vi "Initiate multi-module assembly.vi"(0 "Database Entry in":refnum<class "Database Entry.lvclass">, 11 "error in (no error)":errorcluster) -> (2 "Feet check":bool, 4 "Database Entry out":refnum<class "Database Entry.lvclass">, 6 "Module?":bool, 8 "Abort out":bool, 14 "Module type out":string, 15 "error out":errorcluster)   [LabVIEW 2021, in "Database Entry.lvclass"]
uses:
  Database Entry.lvclass
  Database Entry.lvclass/Database Entry.ctl
  Components/Stack/Stack.lvclass
  <vilib>/Utility/file.llb/Read Delimited Spreadsheet (string).vi
  SubVIs/assembly_tray_region.vi
panel:
  in  "De/Select All":bool
  in  "Set default module type":bool
  out "Now assembling...":string
  in  "Abort":bool
  in  "Relative humidity":dbl
  in  "Temperature (C)":dbl
  in  "Adhesive":u16(ring) items=["Hybrid", "Transfer tape only", "Epoxy only"]
  in  "Module Type":u16(ring) items=["CMU,LD,Full,200,CuW", "CMU,LD,Full,300,CuW", "CMU,LD,Full,300,Ti", "CMU,LD,Full,200,CF", "CMU,LD,Full,300,CF"]
  in  "Operator":u16(ring) items=["jestein", "japicard", "simurthy", "shapoval", "novak", "cmumac"]
  in  "Select positions for assembly":cluster{"1":bool, "2":bool, "3":bool, "4":bool}
  in  "Submit":bool
  # "Tray Slot 1"
  # "Tray Slot 2"
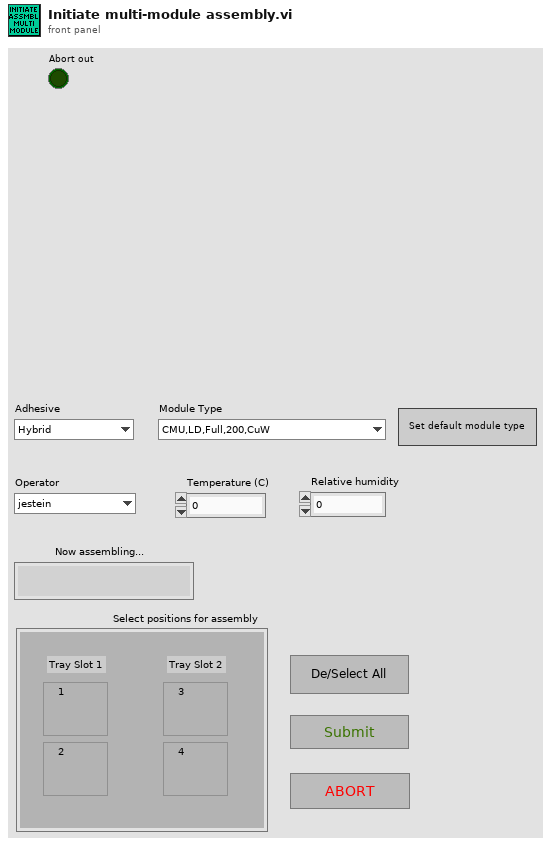
[diagram p1: front panel]
types:
  T1 = typedef "File Paths.ctl" = cluster{"Glue Pattern Folder":path, "Carrier Tray Folder":path, "Pick Up Tool Fixture Folder":path, "Components Folder":path, "Bellows Tool Offset.txt":path, "Pick Up Tool Offset.txt":path, "Dispense Tip Offset.txt":path, "Log Files":path, "Gantry Assembly Map.txt":path, "Syringe and offset map.txt":path, "Controllers Folder":path, "Local dbase config":path}
  T2 = cluster{"[0]":bool, "[1]":bool, "[2]":bool, "[3]":bool}
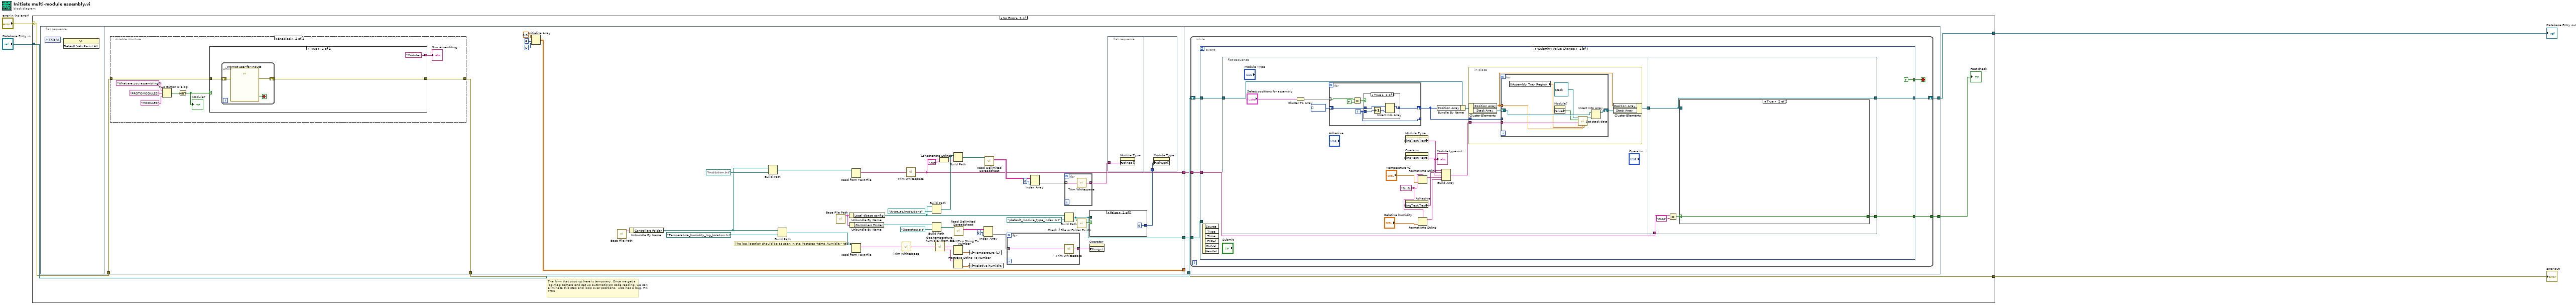
[diagram p0: block diagram]
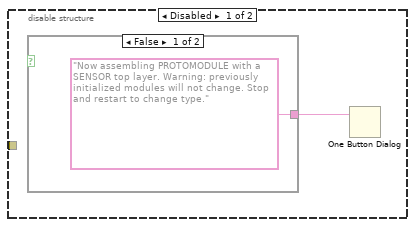
[diagram p2: hidden frame]
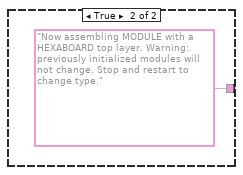
[diagram p3: hidden frame]
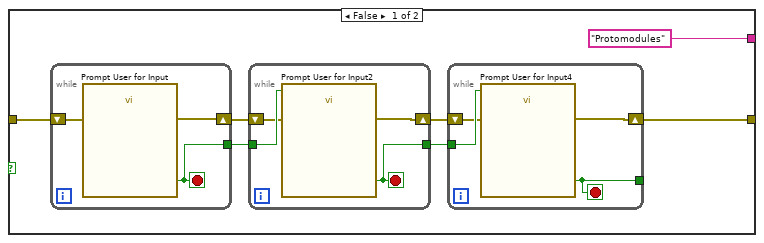
[diagram p4: hidden frame]
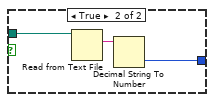
[diagram p5: hidden frame]
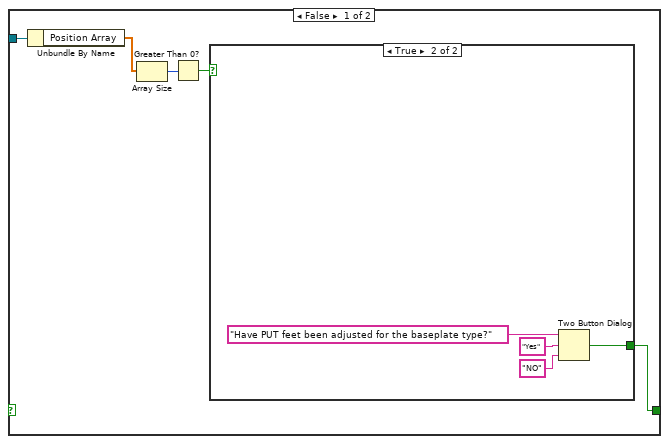
[diagram p7: hidden frame]
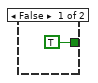
[diagram p8: hidden frame]
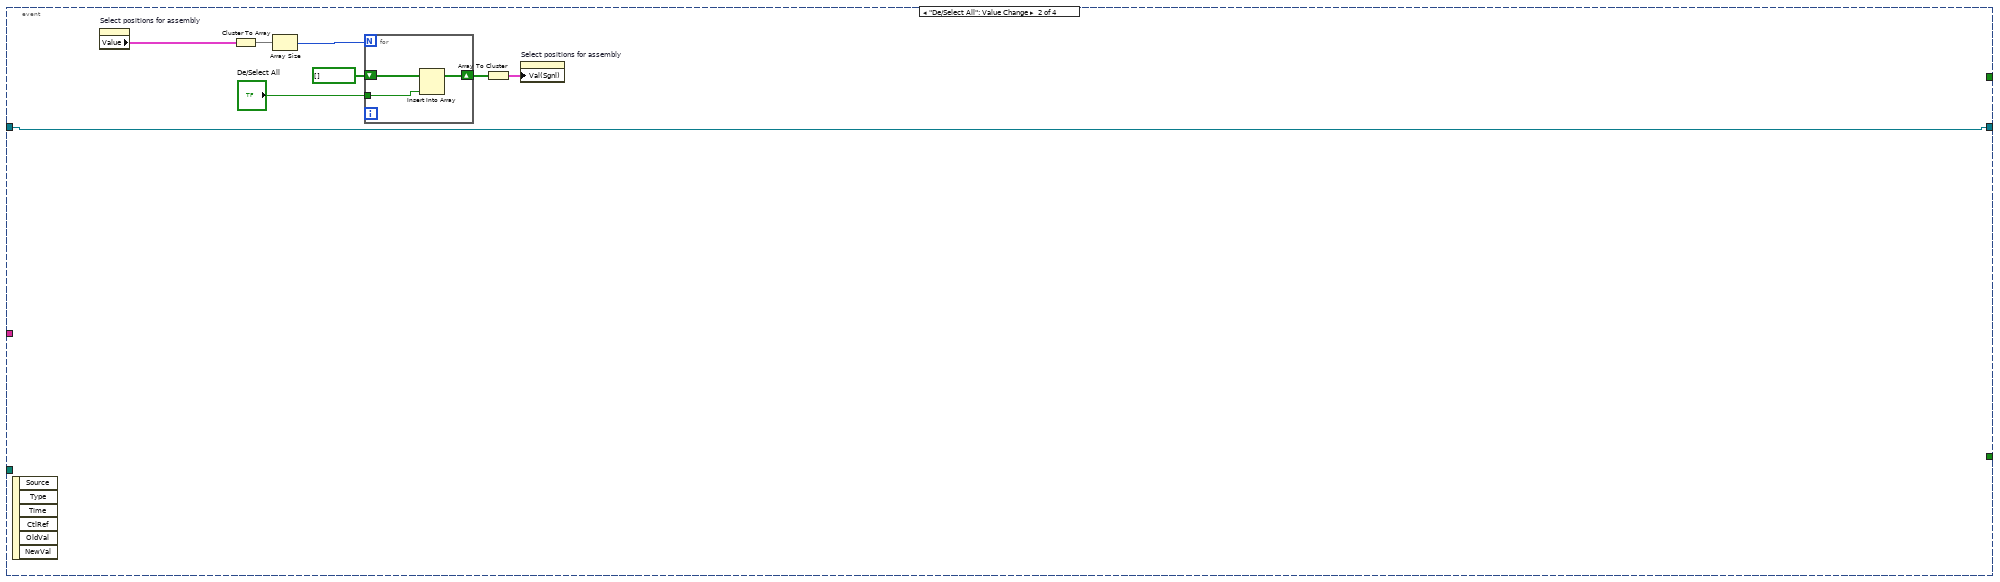
[diagram p9: hidden frame]
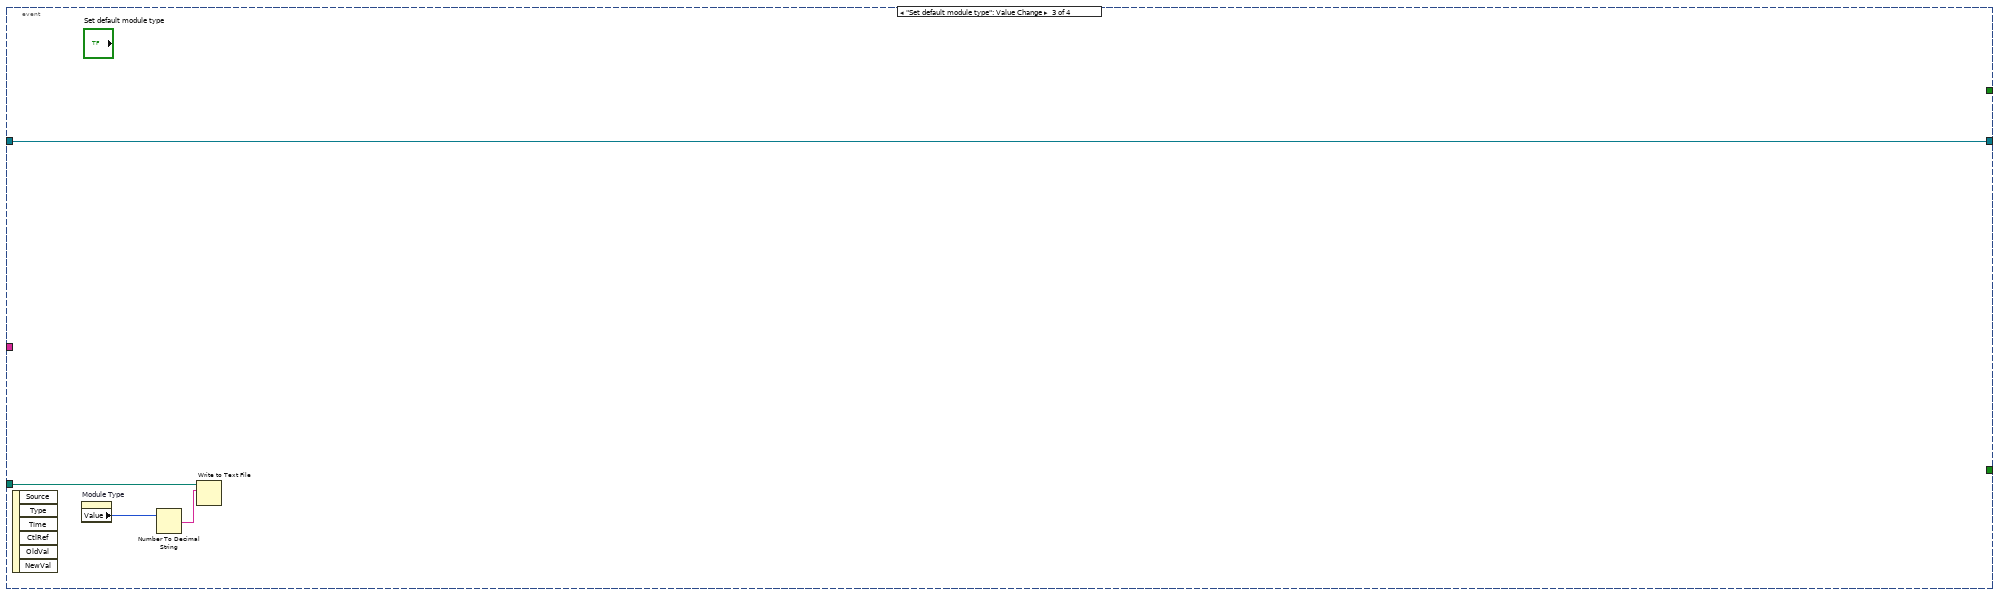
[diagram p10: hidden frame]
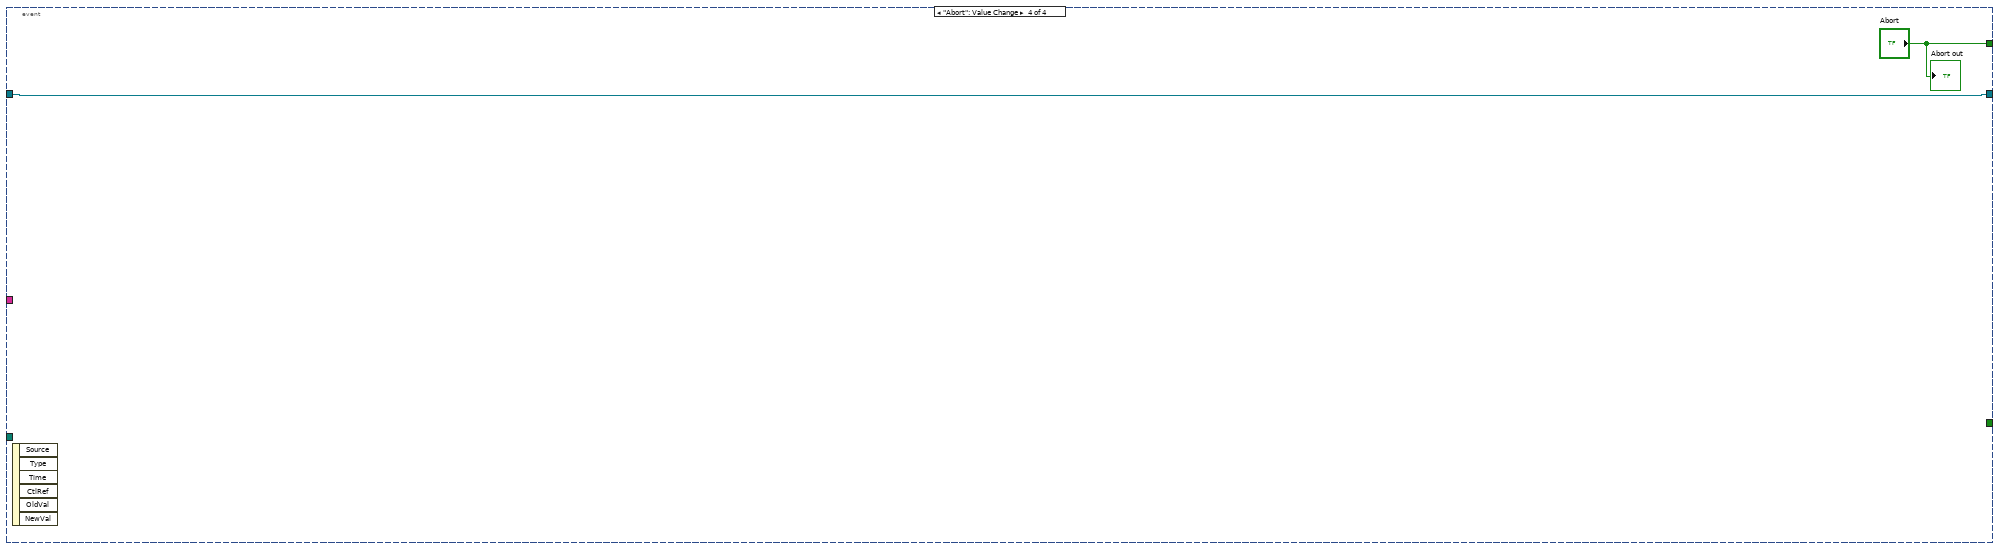
[diagram p11: hidden frame]
diagram:
  n1 = case shown="No Error" "error in (no error)" {
    selector: "error in (no error)" -> [w9 w192]
    tunnel: [w8 w192] -> w3
    tunnel: [w10 w191] -> w1
    tunnel: "Database Entry in" -> [w12 w191]
    frame No Error {
      # "The form that pops up here is temporary. Once we get a log-mag camera and set up automatic QR code reading, we can eliminate this step and loop over positions.  Also has a bug. FIX THIS"
      n2 = flat-sequence {
        tunnel: [w48] -> w7
        tunnel: [w26] -> w6
        tunnel: [w16] -> w5
        tunnel: w9 -> [w15]
        tunnel: [w14] -> w8
        tunnel: w7 -> [_]
        tunnel: w12 -> [w105]
        tunnel: [w104] -> w10
        tunnel: [w103] -> w11
        tunnel: w6 -> [w102]
        tunnel: w5 -> [w101]
        frame #0 {
          n3 = control-ref of="This VI"() -> (w13:refnum<vi>)
          n4 = invoke class="VI" method="Default Vals.Reinit All"(reference=w13) -> ()  [unwired: 2 in, 3 out]
        }
        frame #1 {
          # "The log_location should be as seen in the Postgres \"temp_humidity\" table"
          n5 = disable-structure shown="Enabled" {
            disable-tunnel: w15 -> [_ w60]
            disable-tunnel: [_ w59] -> w14
            frame Disabled {
              n6 = case shown="False" {
                selector: _ -> [_ _]
                tunnel: ["Now assembling PROTOMODULE with a SENSOR top layer. Warning: previously initialized modules will not change. Stop and restart to change type." "Now assembling MODULE with a HEXABOARD top layer. Warning: previously initialized modules will not change. Stop and restart to change type."] -> w56
                frame False {
                }
                frame True {
                }
              }
              n7 = One Button Dialog(message=w56) -> ()  [unwired: 1 in, 1 out]
            }
            frame Enabled {
              n8 = Two Button Dialog(message="What are you assembling?", 1:"MODULES" ("F button name (\"Cancel\")"), 2:"PROTOMODULES" ("T button name (\"OK\")")) -> (T button?=w63:bool)
              n9 = Not(x=w63) -> (.not. x?=w62:bool)
              "Module?" <- w62
              n10 = case shown="True" w62 {
                tunnel: ["Protomodules" ("Now assembling...") "Modules" ("Now assembling...")] -> w61
                tunnel: w60 -> [w68 w85]
                tunnel: [w67 w86] -> w59
                frame False {
                  n11 = while {
                    tunnel: [w84] -> w72
                    shift-right: [w83] -> w70
                    shift-left: w68 -> [w82]
                    stop <- w84 stop-if-true
                    n12 = call "Prompt User for Input"("error in (no error)"=w82) -> ("BPs ready?"=w84:bool, "error out"=w83:errorcluster)  [unwired: 16 in, 1 out]
                  }
                  n13 = while {
                    tunnel: w72 -> [w81]
                    tunnel: [w80] -> w71
                    shift-right: [w78] -> w69
                    shift-left: w70 -> [w79]
                    stop <- w80 stop-if-true
                    n14 = call "Prompt User for Input2"("Enable"=w81, "error in (no error)"=w79) -> ("Sensor tooling ready?"=w80:bool, "error out"=w78:errorcluster)  [unwired: 15 in, 1 out]
                  }
                  n15 = while {
                    tunnel: [w77] -> _
                    tunnel: w71 -> [w76]
                    shift-right: [w74] -> w67
                    shift-left: w69 -> [w75]
                    stop <- w77 stop-if-true
                    n16 = call "Prompt User for Input4"("Enable"=w76, "error in (no error)"=w75) -> ("No gaps?"=w77:bool, "error out"=w74:errorcluster)  [unwired: 15 in, 1 out]
                  }
                }
                frame True {
                  n17 = while {
                    shift-right: [w89] -> w86
                    shift-left: w85 -> [w88]
                    stop <- w90 stop-if-true
                    n18 = call "Prompt User for Input3"("error in (no error)"=w88) -> ("HB tooling ready?"=w90:bool, "error out"=w89:errorcluster)  [unwired: 16 in, 1 out]
                  }
                }
              }
              "Now assembling..." <- w61
            }
          }
          n19 = Initialize Array(0.0 ("element"), 6 ("dimension size"), 6 ("dimension size")) -> (w48:dbl[][])
          n20 = call "Base File Path.vi"() -> ("Paths Out"=w55:T1)  [unwired: 11 in]
          n21 = Unbundle By Name(w55) -> ("Controllers Folder"=w21:path)
          n22 = Build Path(base path=w21, name or relative path=path "Institution.txt") -> (appended path=w32:path)
          n23 = Build Path(base path=w21, name or relative path=path "Temperature_humidity_log_location.txt") -> (appended path=w24:path)
          n24 = call "Base File Path.vi"() -> ("Paths Out"=w44:T1)  [unwired: 11 in]
          n25 = Unbundle By Name(w44) -> ("Local dbase config"=w28:path)
          n26 = Unbundle By Name(w44) -> ("Controllers Folder"=w53:path)
          n27 = Read from Text File(file (use dialog)=w32) -> (text=w34:string)  [unwired: 3 in, 3 out]
          n28 = Read from Text File(file (use dialog)=w24) -> (text=w23:string)  [unwired: 3 in, 3 out]
          n29 = call <vilib>:"Trim Whitespace.vi"("string"=w23) -> ("trimmed string"=w22:string)  [unwired: 1 in]
          n30 = call <vilib>:"Trim Whitespace.vi"("string"=w34) -> ("trimmed string"=w16:string)  [unwired: 1 in]
          n31 = Build Path(base path=w28, name or relative path=path "../type_at_institutions") -> (appended path=w41:path)
          n32 = Build Path(base path=w53, name or relative path=path "Operators.txt") -> (appended path=w51:path)
          n33 = call "Get_temperature_humidity_from_DB.vi"("log_location"=w22) -> ("temp_c"=w20:string, "rel_hum"=w18:string)  [unwired: 1 out]
          n34 = Concatenate Strings(w16, ".txt" ("string")) -> (w39:string)
          n35 = Build Path(base path=w41, name or relative path=w39) -> (appended path=w31:path)
          n36 = Fract/Exp String To Number(string=w20) -> (number=w19:dbl)  [unwired: 3 in, 1 out]
          n37 = Fract/Exp String To Number(string=w18) -> (number=w17:dbl)  [unwired: 3 in, 1 out]
          n38 = call-poly <vilib>:"Read Delimited Spreadsheet.vi"("file path (dialog if empty)"=w51) -> ("all rows"=w50:string[][])  [unwired: 9 in, 5 out]
          n39 = local write "Temperature (C)"(w19) -> ()
          n40 = local write "Relative humidity"(w17) -> ()
          n41 = Index Array(array=w50, index (col)=0 ("disabled index (col)")) -> (element=w37:string[])  [unwired: 1 in]
          n42 = call-poly <vilib>:"Read Delimited Spreadsheet.vi"("file path (dialog if empty)"=w31) -> ("all rows"=w38:string[][])  [unwired: 9 in, 5 out]
          n43 = for {
            tunnel: w37 -> [w100] mode=indexing
            tunnel: [w99] -> w36 mode=indexing
            n44 = call <vilib>:"Trim Whitespace.vi"("string"=w100) -> ("trimmed string"=w99:string)  [unwired: 1 in]
          }
          n45 = Index Array(array=w38, index (col)=0 ("disabled index (col)")) -> (element=w30:string[])  [unwired: 1 in]
          n46 = for {
            tunnel: w30 -> [w98] mode=indexing
            tunnel: [w97] -> w35 mode=indexing
            n47 = call <vilib>:"Trim Whitespace.vi"("string"=w98) -> ("trimmed string"=w97:string)  [unwired: 1 in]
          }
          n48 = Build Path(base path=w28, name or relative path=path "../default_module_type_index.txt") -> (appended path=w26:path)
          n49 = call <vilib>:"Check if File or Folder Exists.vi"("path"=w26) -> ("file or folder exists?"=w29:bool)  [unwired: 8 in, 2 out]
          n50 = case shown="False" w29 {
            tunnel: w26 -> [_ w94]
            tunnel: [0 w92] -> w33
            frame False {
            }
            frame True {
              n51 = Read from Text File(file (use dialog)=w94) -> (text=w93:string)  [unwired: 3 in, 3 out]
              n52 = Decimal String To Number(string=w93) -> (number=w92:i32)  [unwired: 2 in, 1 out]
            }
          }
          n53 = property on="Operator" class="Ring (strict)"("Strings []"=w36) -> ()  [unwired: 2 in, 2 out]
          n54 = flat-sequence {
            tunnel: w35 -> [w95]
            tunnel: w33 -> [w96]
            frame #0 {
              n55 = property on="Module Type" class="Ring (strict)"("Strings []"=w95) -> ()  [unwired: 2 in, 2 out]
            }
            frame #1 {
              n56 = property on="Module Type" class="Ring (strict)"("Val(Sgnl)"=w96) -> ()  [unwired: 2 in, 2 out]
            }
          }
        }
        frame #2 {
          n57 = while {
            shift-right: [w111] -> w104
            shift-left: w105 -> [w110]
            tunnel: [w108] -> w103
            tunnel: w102 -> [w107]
            tunnel: w101 -> [w106]
            stop <- w109 stop-if-true
            n58 = event shown="[0] \"Submit\": Value Change" {
              selector: _ -> [_ _ _ _]
              dyn-events: _ -> [_ _ _ _]
              timeout: _ -> [_ _ _ _]
              tunnel: [TRUE ("T button?") _ _ "Abort"] -> w109
              tunnel: w110 -> [w115 w174 w188 w189]
              tunnel: [w113 w174 w188 w189] -> w111
              tunnel: [w116 _ _ _] -> w108
              tunnel: w107 -> [_ _ w185 _]
              tunnel: w106 -> [w112 _ _ _]
              event "Submit": Value Change {
                n59 = event-data() -> ()  [unwired: 1 in, 6 out]
                n60 = flat-sequence {
                  tunnel: w115 -> [w130]
                  tunnel: [w125] -> w114
                  tunnel: [w162] -> w116
                  tunnel: w114 -> [w161]
                  tunnel: [w161] -> w113
                  tunnel: w112 -> [w159]
                  frame #0 {
                    w118 = "%.;%f" ("format string")
                    n61 = Cluster To Array(cluster="Select positions for assembly") -> (array=w133:bool[])
                    n62 = for {
                      shift-right: [w149] -> w127
                      shift-left: i32[] [] -> [w150]
                      tunnel: [w148] -> _
                      tunnel: w133 -> [w147] mode=indexing
                      i -> [w148]
                      n63 = Equal?(x=w147, y=TRUE) -> (x = y?=w151:bool)
                      n64 = case shown="True" w151 {
                        tunnel: w150 -> [w153 w156]
                        tunnel: w148 -> [_ w155]
                        tunnel: [w153 w154] -> w149
                        frame False {
                        }
                        frame True {
                          n65 = Increment(x=w155) -> (x+1=w157:i32)
                          n66 = Insert Into Array(array=w156, new element=w157) -> (w154:i32[])  [unwired: 1 in]
                        }
                      }
                    }
                    n67 = property on="Module Type" class="Ring (strict)"() -> ("RingText.Text"=w123:string)  [unwired: 2 in, 2 out]
                    "Module type out" <- w123
                    n68 = property on="Operator" class="Ring (strict)"() -> ("RingText.Text"=w129:string)  [unwired: 2 in, 2 out]
                    n69 = property on="Adhesive" class="Ring (strict)"() -> ("RingText.Text"=w128:string)  [unwired: 2 in, 2 out]
                    n70 = Format Into String(format string=w118, "Temperature (C)") -> (resulting string=w121:string)  [unwired: 2 in, 1 out]
                    n71 = Format Into String(format string=w118, "Relative humidity") -> (resulting string=w119:string)  [unwired: 2 in, 1 out]
                    n72 = Bundle By Name(cluster=w130, "Position Array"=w127) -> (w126:refnum<class "Database Entry.lvclass">)
                    n73 = Build Array(w123, w128, w129, w121, w119) -> (w124:string[])
                    n74 = in-place {
                      in-place-border: w127 -> [w138]
                      in-place-border: w124 -> [w135]
                      n75 = in-place-cluster #1(w126) -> ("Position Array"=w134:dbl[], "Stack Array"=w137:refnum<class "Stack.lvclass">[])
                      n76 = for {
                        tunnel: w138 -> [_] mode=indexing
                        shift-right: [w145] -> w136
                        shift-left: w137 -> [w146]
                        tunnel: w135 -> [w142]
                        tunnel: w134 -> [w140] mode=indexing
                        n77 = global read "assembly_tray_region.vi" "Assembly Tray Region"() -> (w139:dbl)
                        n78 = property on="Module?" class="Bool (strict)"() -> ("Value"=w141:bool)  [unwired: 2 in, 2 out]
                        n79 = call "Set stack data.vi"("Region"=w139, "Position"=w140, "Common data array"=w142, "Is module?"=w141, "Stack in"=refnum<class "Stack.lvclass"> refnum ("Stack.lvclass")) -> ("Stack out"=w143:refnum<class "Stack.lvclass">)  [unwired: 5 in, 1 out]
                        n80 = Insert Into Array(array=w146, new element=w143) -> (w145:refnum<class "Stack.lvclass">[])  [unwired: 1 in]
                      }
                      n81 = in-place-cluster #1("Position Array"=w134, "Stack Array"=w136) -> (w125:refnum<class "Database Entry.lvclass">)
                    }
                  }
                  frame #1 {
                    n82 = Equal?(x=w159, y="CMU") -> (x = y?=w160:bool)
                    n83 = case shown="True" w160 {
                      selector: w160 -> [_ w173]
                      tunnel: [w167 w173] -> w162
                      tunnel: w161 -> [w163 _]
                      frame False {
                        n84 = Unbundle By Name(w163) -> ("Position Array"=w166:dbl[])
                        n85 = Array Size(array=w166) -> (size(s)=w165:i32)
                        n86 = Greater Than 0?(x=w165) -> (x > 0?=w164:bool)
                        n87 = case shown="True" w164 {
                          tunnel: [TRUE ("T button?") w169] -> w167
                          frame False {
                          }
                          frame True {
                            n88 = Two Button Dialog(message="Have PUT feet been adjusted for the baseplate type?", 1:"NO" ("F button name (\"Cancel\")"), 2:"Yes" ("T button name (\"OK\")")) -> (T button?=w169:bool)
                          }
                        }
                      }
                      frame True {
                      }
                    }
                  }
                }
              }
              event "De/Select All": Value Change {
                n89 = event-data() -> ()  [unwired: 1 in, 6 out]
                n90 = property on="Select positions for assembly" class="Clust (strict)"() -> ("Value"=w181:cluster{"1":bool, "2":bool, "3":bool, "4":bool})  [unwired: 2 in, 2 out]
                n91 = Cluster To Array(cluster=w181) -> (array=w180:bool[])
                n92 = Array Size(array=w180) -> (size(s)=w179:i32)
                n93 = for {
                  N: w179 -> [_]
                  shift-right: [w183] -> w177
                  shift-left: bool[] [] -> [w184]
                  tunnel: "De/Select All" -> [w182]
                  n94 = Insert Into Array(array=w184, new element=w182) -> (w183:bool[])  [unwired: 1 in]
                }
                n95 = Array To Cluster(array=w177) -> (cluster=w176:T2)
                n96 = property on="Select positions for assembly" class="Clust (strict)"("Val(Sgnl)"=w176) -> ()  [unwired: 2 in, 2 out]
              }
              event "Set default module type": Value Change {
                n97 = event-data() -> ()  [unwired: 1 in, 6 out]
                n98 = property on="Module Type" class="Ring (strict)"() -> ("Value"=w186:u16)  [unwired: 2 in, 2 out]
                n99 = Number To Decimal String(number=w186) -> (decimal integer string=w187:string)  [unwired: 1 in]
                n100 = Write to Text File(file (use dialog)=w185, text=w187) -> ()  [unwired: 2 in, 3 out]
              }
              event "Abort": Value Change {
                n101 = event-data() -> ()  [unwired: 1 in, 6 out]
                "Abort out" <- "Abort"
              }
            }
          }
        }
      }
      "Feet check" <- w11
    }
    frame Error {
    }
  }
  "error out" <- w3
  "Database Entry out" <- w1
